vi "test Pointer Lifecycle.vi"(8 "error in (no error)":errorcluster, 11 "Test Case in":refnum<class "Lifecycle Tests.lvclass">) -> (0 "error out":errorcluster, 3 "Test Case out":refnum<class "Lifecycle Tests.lvclass">)   [LabVIEW 2027, in "Memory Manager Tests.lvlib" / "Lifecycle Tests.lvclass"]
uses:
  Lifecycle Tests.lvclass
  Classes/Pointer/Pointer.lvclass
  C:/Program Files/National Instruments/LabVIEW 2027/vi.lib/addons/_JKI Toolkits/VI Tester/TestCase.llb/TestCase.lvclass
  <vilib>/addons/_JKI Toolkits/VI Tester/TestCase.llb/TestCase.lvclass
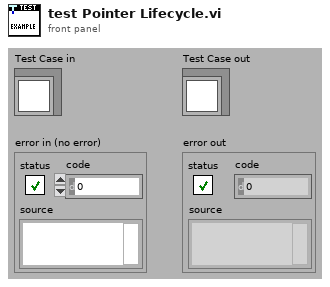
[diagram p1: front panel]
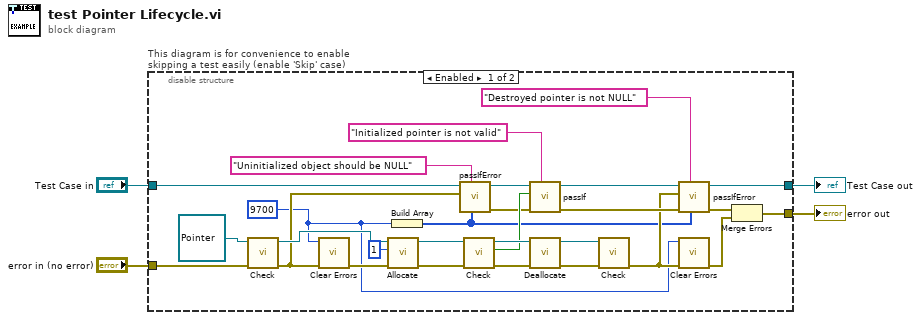
[diagram p0: block diagram]
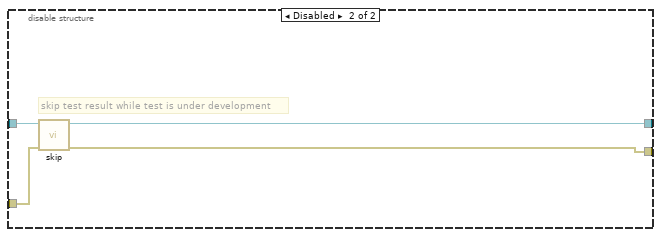
[diagram p2: hidden frame]
diagram:
  n1 = disable-structure "This diagram is for convenience to enable skipping a test easily (enable 'Skip' case)" shown="Enabled" {
    disable-tunnel: "Test Case in" -> [w15 w36]
    disable-tunnel: [w16 w34] -> w2
    disable-tunnel: [w23 w35] -> w1
    disable-tunnel: "error in (no error)" -> [w11 w33]
    frame Enabled {
      w12 = 9700 ("pass error code (0=any error code)")
      n2 = call "Check.vi"("error in (no error)"=w11, "Pointer in"=refnum<class "Pointer.lvclass"> refnum) -> ("error out"=w19:errorcluster, "Pointer out"=w31:refnum<class "Pointer.lvclass">)  [unwired: 7 in, 1 out]
      n3 = call <vilib>:"Clear Errors.vi"("error in (no error)"=w19, "specific error code to clear (0: all)"=w12) -> ("error out"=w18:errorcluster)  [unwired: 4 in, 1 out]
      n4 = call "Allocate.vi"("error in (no error)"=w18, "size"=u64 1, "Pointer type"=w31) -> ("error out"=w29:errorcluster, "Pointer out"=w30:refnum<class "Pointer.lvclass">)  [unwired: 7 in]
      n5 = Build Array(w12) -> (w13:i32[])
      n6 = call-dynamic "passIfError.vi"("passing error codes (default = any error code)"=w13, "custom report message (\"\")"="Uninitialized object should be NULL" ("task (\"\")"), "error"=w19, "TestCase in"=w15) -> ("error out"=w26:errorcluster, "TestCase out"=w14:refnum<class "Lifecycle Tests.lvclass">)  [unwired: 6 in]
      n7 = call "Check.vi"("error in (no error)"=w29, "Pointer in"=w30) -> ("error out"=w9:errorcluster, "LabVIEW pointer?"=w27:bool, "Pointer out"=w28:refnum<class "Pointer.lvclass">)  [unwired: 7 in]
      n8 = call-dynamic "passIf.vi"("custom report message (\"\")"="Initialized pointer is not valid" ("task (\"\")"), "error in (no error)"=w26, "pass"=w27, "TestCase in"=w14) -> ("error out"=w25:errorcluster, "TestCase out"=w17:refnum<class "Lifecycle Tests.lvclass">)  [unwired: 6 in]
      n9 = call "Deallocate.vi"("error in (no error)"=w9, "Pointer"=w28) -> ("error out"=w20:errorcluster, "Pointer type"=w21:refnum<class "Pointer.lvclass">)  [unwired: 8 in]
      n10 = call "Check.vi"("error in (no error)"=w20, "Pointer in"=w21) -> ("error out"=w22:errorcluster)  [unwired: 7 in, 2 out]
      n11 = call-dynamic "passIfError.vi"("passing error codes (default = any error code)"=w13, "custom report message (\"\")"="Destroyed pointer is not NULL" ("task (\"\")"), "error in (no error)"=w25, "error"=w22, "TestCase in"=w17) -> ("error out"=w24:errorcluster, "TestCase out"=w16:refnum<class "Lifecycle Tests.lvclass">)  [unwired: 5 in]
      n12 = call <vilib>:"Clear Errors.vi"("error in (no error)"=w22, "specific error code to clear (0: all)"=w12) -> ("error out"=w10:errorcluster)  [unwired: 4 in, 1 out]
      n13 = Merge Errors(w24, w10) -> (w23:errorcluster)
    }
    frame Disabled {
      # "skip test result while test is under development"
      n14 = call <vilib>:"skip.vi"("error in (no error)"=w33, "TestCase in"=w36) -> ("error out"=w35:errorcluster, "TestCase out"=w34:refnum<class "Lifecycle Tests.lvclass">)  [unwired: 8 in]
    }
  }
  "error out" <- w1
  "Test Case out" <- w2
